vi "Read resolution.vi"(8 "error in (no error)":errorcluster, 11 "VISA resource name":refnum<visa-resource-name>) -> (0 "error out":errorcluster, 2 "Resolution":string, 3 "VISA resource name out":refnum<visa-resource-name>)   [LabVIEW 2021, in "Ceyear.lvlib"]
doc: "Reads a trace from the spectrum analyzer."
uses:
  <instrlib>/Ceyear/Ceyear.lvlib
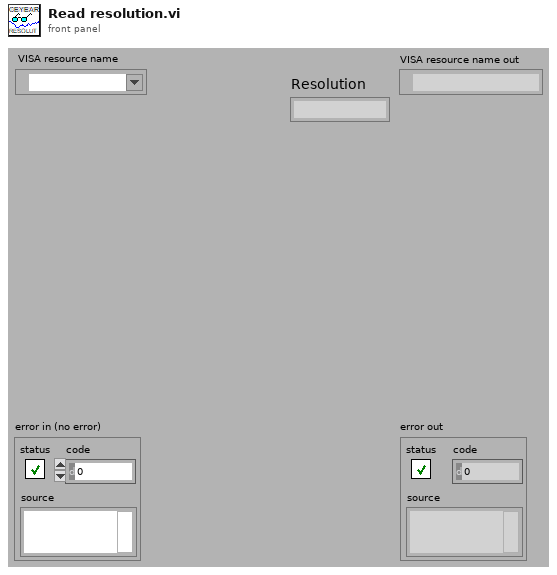
[diagram p1: front panel]
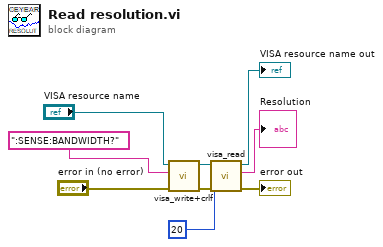
[diagram p0: block diagram]
diagram:
  n1 = call <instrlib>:"visa_write+crlf.vi"("error in (no error)"="error in (no error)", "Strings (empty)"=":SENSE:BANDWIDTH?" ("write buffer"), "VISA resource name"="VISA resource name") -> ("error out"=w8:errorcluster, "VISA resource name out"=w9:refnum<visa-resource-name>)  [unwired: 7 in]
  n2 = call <instrlib>:"visa_read.vi"("error in (no error)"=w8, "Byte Count (0)"=u32 20, "VISA resource name"=w9) -> ("error out"=→"error out":errorcluster, "Read Data"=→"Resolution":string, "VISA resource name out"=→"VISA resource name out":refnum<visa-resource-name>)  [unwired: 5 in, 1 out]
